vi "Write Include Invalid Names.vi"(8 "error in (no error)":errorcluster, 10 "IncludeInvalidNames":bool, 11 "DAQmxName.lvclass in":refnum<class "DAQmxName.lvclass">) -> (0 "error out":errorcluster, 3 "DAQmxName.lvclass out":refnum<class "DAQmxName.lvclass">)   [LabVIEW 2015, in "DAQmxName.lvclass"]
uses:
  DAQmxName.lvclass
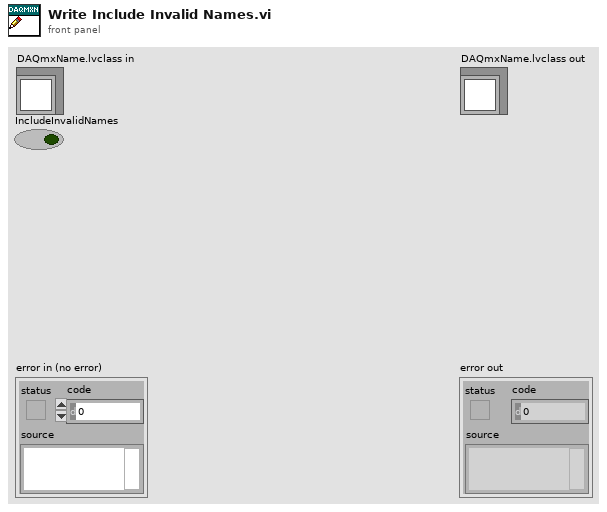
[diagram p1: front panel]
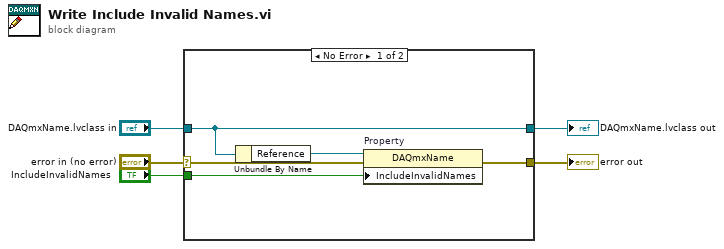
[diagram p0: block diagram]
diagram:
  n1 = case shown="No Error" "error in (no error)" {
    selector: "error in (no error)" -> [w6 w12]
    tunnel: [w10 w12] -> w4
    tunnel: [w8 w11] -> w2
    tunnel: "DAQmxName.lvclass in" -> [w8 w11]
    tunnel: "IncludeInvalidNames" -> [w9 _]
    frame No Error {
      n2 = Unbundle By Name(w8) -> ("Reference"=w7:refnum<vi>)
      n3 = property on="Property" class="DAQmxName"(reference=w7, error in=w6, "IncludeInvalidNames"=w9) -> (error out=w10:errorcluster)  [unwired: 1 out]
    }
    frame Error {
    }
  }
  "error out" <- w4
  "DAQmxName.lvclass out" <- w2
